vi "Get XY Graph Plot Names.vi"(8 "error in (no error)":errorcluster, 11 "graph_utilities in":refnum<class "graph_utilities.lvclass">) -> (0 "error out":errorcluster, 2 "Plot Names []":string[](array[string]), 3 "graph_utilities out":refnum<class "graph_utilities.lvclass">)   [LabVIEW 2020, in "graph_utilities.lvclass"]
doc: "Get all plot names."
uses:
  graph_utilities.lvclass
  graph_utilities.lvclass/graph_utilities.ctl
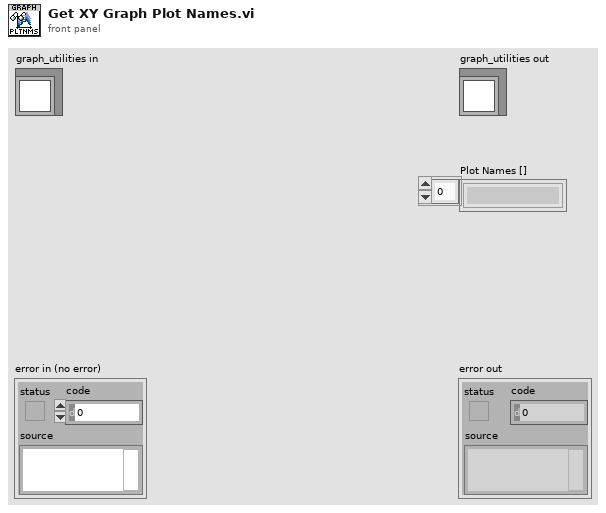
[diagram p1: front panel]
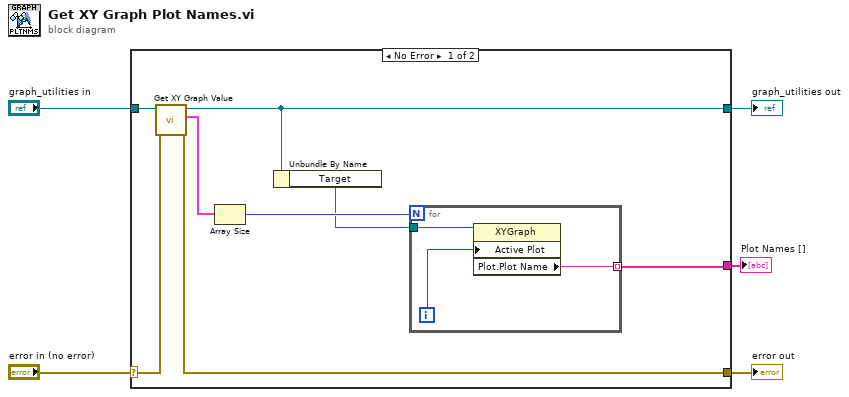
[diagram p0: block diagram]
diagram:
  n1 = case shown="No Error" "error in (no error)" {
    selector: "error in (no error)" -> [w12 w18]
    tunnel: [w9 w18] -> w4
    tunnel: [w11 w17] -> w2
    tunnel: "graph_utilities in" -> [w13 w17]
    tunnel: [w6 _] -> w1
    frame No Error {
      n2 = call "Get XY Graph Value.vi"("error in (no error)"=w12, "graph_utilities in"=w13) -> ("error out"=w9:errorcluster, "Value"=w8:cluster{"X":dbl[], "Y":dbl[]}[], "graph_utilities out"=w11:refnum<class "graph_utilities.lvclass">)  [unwired: 7 in]
      n3 = Array Size(array=w8) -> (size(s)=w10:i32)
      n4 = Unbundle By Name(w11) -> ("Target"=w7:refnum<vi>)
      n5 = for {
        N: w10 -> [_]
        tunnel: w7 -> [w15]
        tunnel: [w14] -> w6 mode=indexing
        i -> [w16]
        n6 = property on="Property Node" class="XYGraph"(reference=w15, "Active Plot"=w16) -> ("Plot.Plot Name"=w14:string)  [unwired: 1 in, 2 out]
      }
    }
    frame Error {
    }
  }
  "error out" <- w4
  "graph_utilities out" <- w2
  "Plot Names []" <- w1
